vi "WLAN_SendOnce.vi"(8 "error in (no error)":errorcluster, 10 "data":cdb[](array[numeric]), 11 "session handle":refnum<k15>) -> (0 "error out":errorcluster)   [LabVIEW 2014]
uses:
  <instrlib>/niUSRP/niUSRP Write Tx Data (CDB).vi
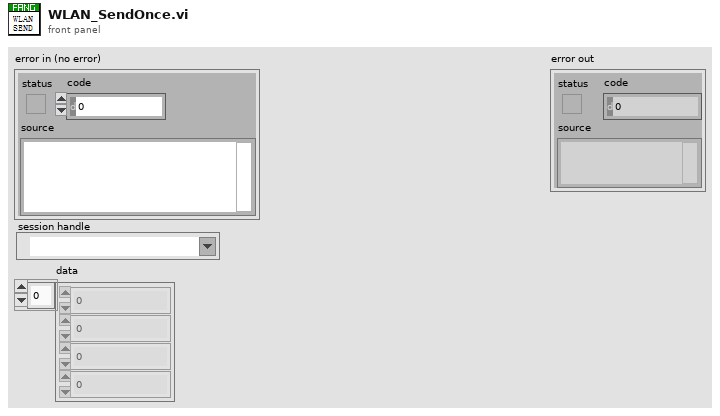
[diagram p1: front panel]
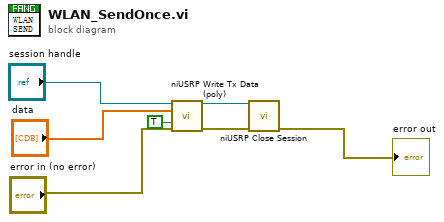
[diagram p0: block diagram]
diagram:
  n1 = call-poly <instrlib>:"niUSRP Write Tx Data (poly).vi"("session handle"="session handle", "data"="data", "end of data?"=TRUE, "error in (no error)"="error in (no error)") -> ("session handle out"=w2:refnum<k15>, "error out"=w7:errorcluster)  [unwired: 10 in]
  n2 = call <instrlib>:"niUSRP Close Session.vi"("session handle"=w2, "error in (no error)"=w7) -> ("error out"=→"error out":errorcluster)  [unwired: 13 in]
